vi "Init I2C.vi"(8 "error in (no error)":errorcluster, 9 "Baud":u32=400000 format="%.0p", 10 "I2C In":T1=-1, 11 "Session in":refnum<class "Session.lvclass">) -> (0 "error out":errorcluster, 3 "Session out":refnum<class "Session.lvclass">)   [LabVIEW 2024, in "CTI.lvlib" / "Session.lvclass"]
uses:
  Session.lvclass
  I2C Number.ctl
  DeviceComms/DeviceComms.lvclass
  I2C/I2C.lvclass
  CTI.lvlib
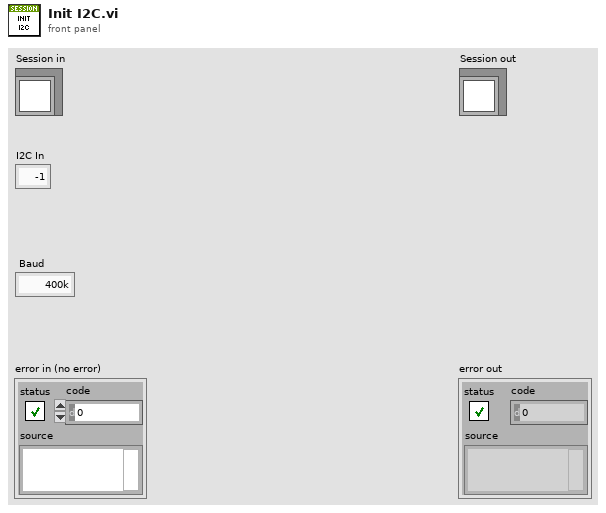
[diagram p1: front panel]
types:
  T1 = typedef "CTI.lvlib/I2C Number.ctl" = i8
  T2 = typedef "CTI.lvlib/GPIO Number.ctl" = i8
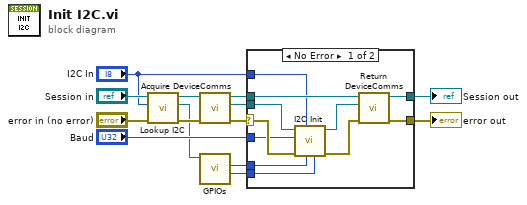
[diagram p0: block diagram]
diagram:
  n1 = call "Lookup I2C.vi"("error in (no error)"="error in (no error)", "I2C #"="I2C In", "Session in"="Session in") -> ("error out"=w5:errorcluster, "I2C"=w1:refnum<class "I2C.lvclass">, "Session out"=w3:refnum<class "Session.lvclass">)  [unwired: 6 in]
  n2 = call "Acquire DeviceComms.vi"("error in (no error)"=w5, "Session in"=w3) -> ("error out"=w14:errorcluster, "DeviceComms"=w10:refnum<class "DeviceComms.lvclass">, "Session out"=w11:refnum<class "Session.lvclass">)  [unwired: 7 in]
  n3 = call "GPIOs.vi"("I2C in"=w1) -> ("SDA GPIO"=w8:T2, "SCL GPIO"=w9:T2)  [unwired: 7 in, 2 out]
  n4 = case shown="No Error" w14 {
    selector: w14 -> [w25 w26]
    tunnel: "Baud" -> [w24 _]
    tunnel: w11 -> [w23 w27]
    tunnel: w10 -> [w22 _]
    tunnel: w9 -> [w21 _]
    tunnel: w8 -> [w20 _]
    tunnel: "I2C In" -> [w19 _]
    tunnel: [w18 w27] -> w7
    tunnel: [w15 w26] -> w6
    frame No Error {
      n5 = call-dynamic "I2C Init.vi"("SDA GPIO"=w20, "SCL GPIO"=w21, "I2C #"=w19, "error in (no error)"=w25, "Baud"=w24, "DeviceComms in"=w22) -> ("error out"=w16:errorcluster, "DeviceComms out"=w17:refnum<class "DeviceComms.lvclass">)  [unwired: 4 in]
      n6 = call "Return DeviceComms.vi"("error in (no error)"=w16, "DeviceComms"=w17, "Session in"=w23) -> ("error out"=w15:errorcluster, "Session out"=w18:refnum<class "Session.lvclass">)  [unwired: 7 in]
    }
    frame Error {
    }
  }
  "error out" <- w6
  "Session out" <- w7
